vi "Cycle.vi"() -> ()   [LabVIEW 2011]
doc: "This example is a template that gives the structure of a single-loop PID controller. This VI uses the PID Filter VI to reduce measurement noise. This VI also uses the PID Autotuning VI to tune the controller based on the closed-loop response. This VI also uses the Timed Loop to ensure deterministic execution.\n\nReplace the Dummy Input and Dummy Output VIs with code that communicates with a real-time target."
uses:
  <vilib>/Platform/TimedLoop/XDataNode/timing_clust.ctl
  <vilib>/Platform/TimedLoop/XDataNode/nitl_modes.ctl
  <vilib>/Platform/TimedLoop/XDataNode/wakeup.ctl
  <vilib>/DAQmx/write.llb/DAQmx Write (Digital 1D Bool NChan 1Samp 1Line).vi
  <vilib>/DAQmx/write.llb/DAQmx Write (Counter Frequency 1Chan 1Samp).vi
  <vilib>/DAQmx/create/channels.llb/DAQmx Create Channel (CO-Pulse Generation-Frequency).vi
  <vilib>/DAQmx/configure/timing.llb/DAQmx Timing (Implicit).vi
  <vilib>/DAQmx/miscellaneous.llb/DAQmx Fill In Error Info.vi
  <vilib>/Platform/TimedLoop/XDataNode/XDataNode.xnode
  <vilib>/Platform/TimedLoop/XDataNode/XDNodeRunTimeDep.lvlib
panel:
  in  "duty cycle":dbl=0.8 format="%_6g"
  in  "Period":i64=1000
  in  "Switch":bool
  in  "stop 2":bool
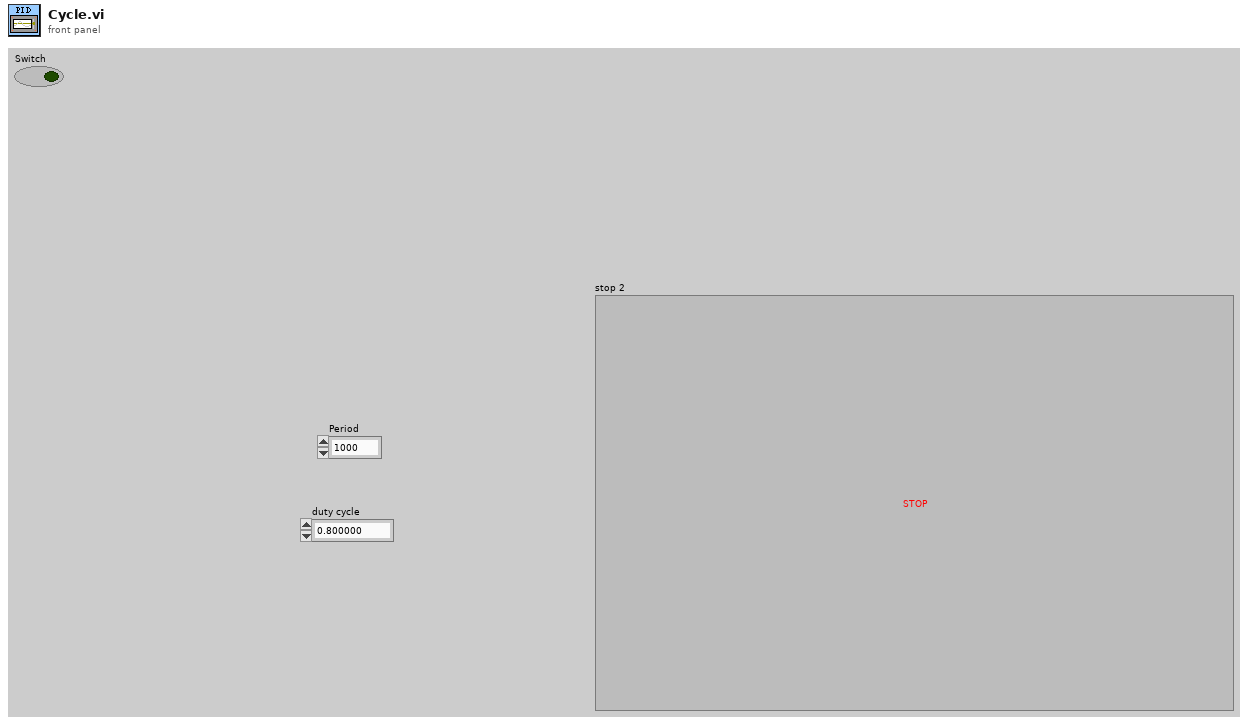
[diagram p1: front panel]
types:
  T1 = typedef "XDNodeRunTimeDep.lvlib/timing_clust.ctl" = cluster{"Expected End [f-1]":u64, "Actual End [f-1]":u64, "Finished Late? [f-1]":bool, "Expected End [i-1]":u64, "Actual End [i-1]":u64, "Finished Late? [i-1]":bool, "Expected Start [i]":u64, "Actual Start [i]":u64, "Expected Start [f]":u64, "Actual Start [f]":u64, "Source Name":string, "Structure Name":string, "Period":i64, "Deadline":i64, "Offset":i64, "Start":i64, "Priority":i32, "Timeout":i32, "Mode":T2, "Wakeup Reason":T3, "Error":errorcluster, "Source Type":string, "Secondary Source Type":string, "Global End Time":u64, "Global Start Time":u64, "Frame Duration":u64, "Iteration Duration":u64, "Assigned CPU":i32, "I/O Scan Engine Mode":u32}
  T2 = typedef "XDNodeRunTimeDep.lvlib/nitl_modes.ctl" = enum32{"No Change", "Process missed periods, maintain original phase", "Discard missed periods, maintain original phase", "Process missed periods, ignore original phase", "Discard missed periods, ignore original phase"}
  T3 = typedef "XDNodeRunTimeDep.lvlib/wakeup.ctl" = enum32{"Normal", "Aborted", "Asynchronous wakeup", "Timing source error", "Timed loop error", "Timeout"}
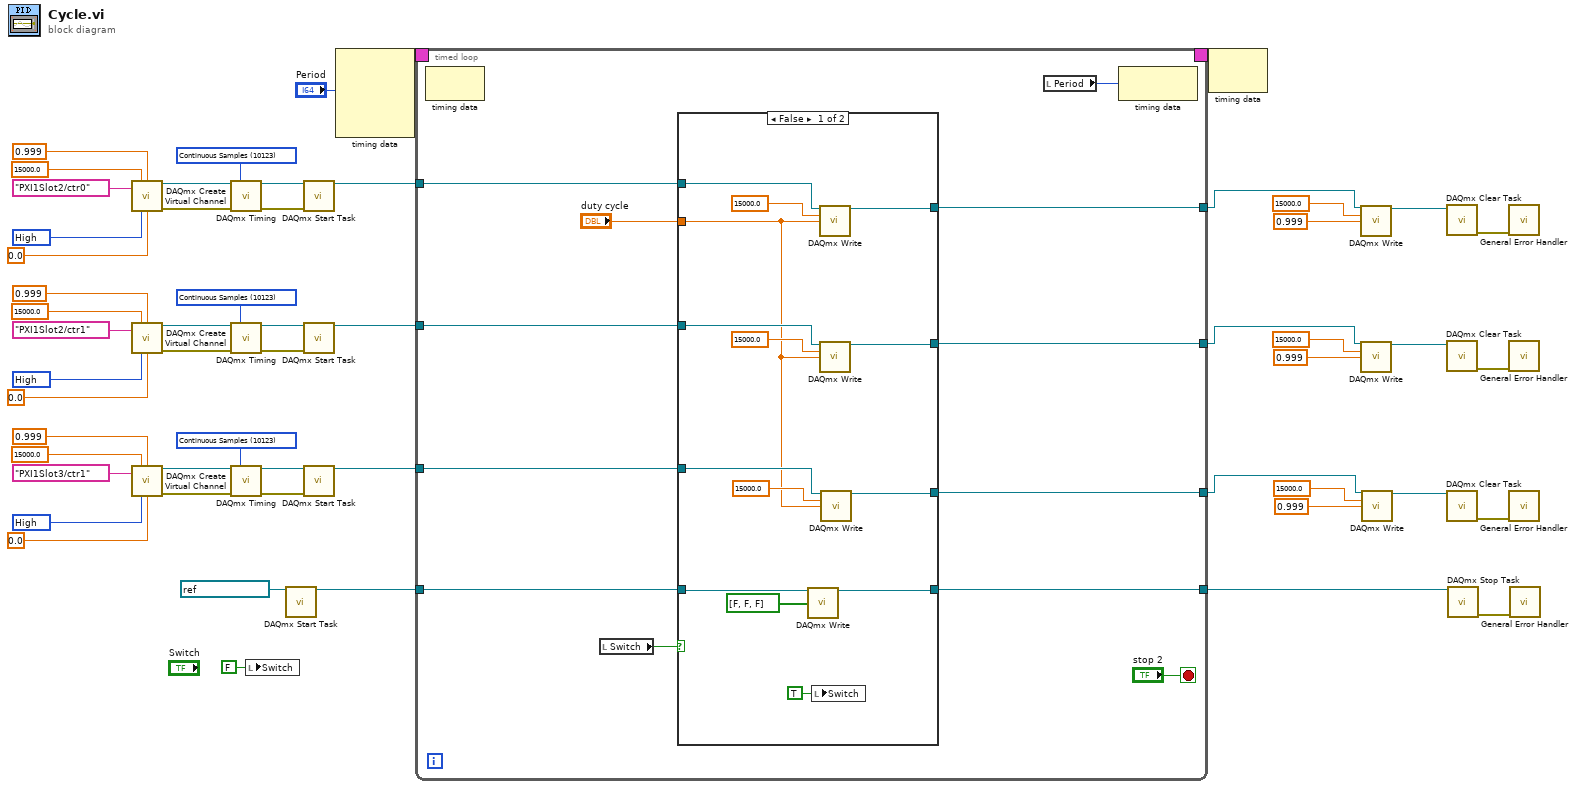
[diagram p0: block diagram]
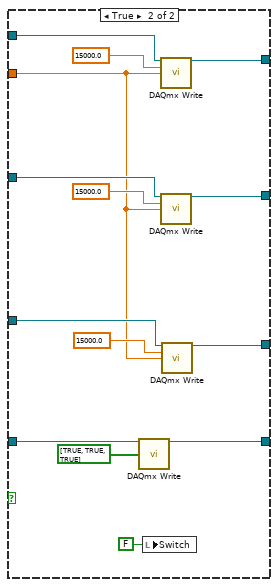
[diagram p2: hidden frame]
diagram:
  w48 = 10192 items=["High"=10192, "Low"=10214] ("idle state")
  w54 = 10123 items=["Finite Samples"=10178, "Continuous Samples"=10123] ("sample mode")
  w41 = 10192 items=["High"=10192, "Low"=10214] ("idle state")
  w35 = 10123 items=["Finite Samples"=10178, "Continuous Samples"=10123] ("sample mode")
  w28 = 10192 items=["High"=10192, "Low"=10214] ("idle state")
  w34 = 10123 items=["Finite Samples"=10178, "Continuous Samples"=10123] ("sample mode")
  n1 = call-poly <vilib>:"DAQmx Create Virtual Channel.vi"("frequency"=15000.0 ("duty cycle"), "duty cycle"=0.999, "counter"=tag "PXI1Slot2/ctr0", "idle state"=w28, "initial delay"=0.0) -> ("task out"=w31:refnum<k21>, "error out"=w30:errorcluster)  [unwired: 9 in]
  n2 = call-poly <vilib>:"DAQmx Create Virtual Channel.vi"("frequency"=15000.0 ("duty cycle"), "duty cycle"=0.999, "counter"=tag "PXI1Slot2/ctr1", "idle state"=w41, "initial delay"=0.0) -> ("task out"=w38:refnum<k21>, "error out"=w39:errorcluster)  [unwired: 9 in]
  n3 = call-poly <vilib>:"DAQmx Create Virtual Channel.vi"("frequency"=15000.0 ("duty cycle"), "duty cycle"=0.999, "counter"=tag "PXI1Slot3/ctr1", "idle state"=w48, "initial delay"=0.0) -> ("task out"=w51:refnum<k21>, "error out"=w50:errorcluster)  [unwired: 9 in]
  n4 = call-poly <vilib>:"DAQmx Timing.vi"("task/channels in"=w31, "sample mode"=w34, "error in"=w30) -> ("task out"=w33:refnum<k21>, "error out"=w32:errorcluster)  [unwired: 11 in]
  n5 = call-poly <vilib>:"DAQmx Timing.vi"("task/channels in"=w38, "sample mode"=w35, "error in"=w39) -> ("task out"=w36:refnum<k21>, "error out"=w37:errorcluster)  [unwired: 11 in]
  n6 = call-poly <vilib>:"DAQmx Timing.vi"("task/channels in"=w51, "sample mode"=w54, "error in"=w50) -> ("task out"=w53:refnum<k21>, "error out"=w52:errorcluster)  [unwired: 11 in]
  n7 = local write "Switch"(FALSE ("Switch")) -> ()
  n8 = call <vilib>:"DAQmx Start Task.vi"("task/channels in"=refnum<k21> "MotorDirABC") -> ("task out"=w16:refnum<k21>)  [unwired: 13 in, 1 out]
  n9 = call <vilib>:"DAQmx Start Task.vi"("task/channels in"=w33, "error in"=w32) -> ("task out"=w21:refnum<k21>)  [unwired: 12 in, 1 out]
  n10 = call <vilib>:"DAQmx Start Task.vi"("task/channels in"=w36, "error in"=w37) -> ("task out"=w20:refnum<k21>)  [unwired: 12 in, 1 out]
  n11 = call <vilib>:"DAQmx Start Task.vi"("task/channels in"=w53, "error in"=w52) -> ("task out"=w19:refnum<k21>)  [unwired: 12 in, 1 out]
  n12 = node-c288("Period") -> (w56:T1)  [unwired: 3 in]
  n13 = timed-loop {
    timing: w56 -> [_]
    timing-out: [_] -> w55
    tunnel: w21 -> [w68]
    tunnel: w20 -> [w67]
    tunnel: w19 -> [w66]
    tunnel: [w64] -> w5
    tunnel: [w63] -> w6
    tunnel: [w62] -> w7
    tunnel: w16 -> [w61]
    tunnel: [w60] -> w15
    stop <- "stop 2" stop-if-true
    n14 = node-c288() -> ()  [unwired: 1 in, 1 out]
    n15 = local read "Switch"() -> (w59:bool)
    n16 = case shown="False" w59 {
      tunnel: w68 -> [w70 w89]
      tunnel: w67 -> [w75 w87]
      tunnel: w66 -> [w73 w85]
      tunnel: [w69 w88] -> w64
      tunnel: [w74 w86] -> w63
      tunnel: [w72 w84] -> w62
      tunnel: w61 -> [w79 w96]
      tunnel: [w80 w95] -> w60
      tunnel: "duty cycle" -> [w71 w83]
      frame False {
        n17 = call-poly <vilib>:"DAQmx Write.vi"("task/channels in"=w79, "data"=bool[] [FALSE, FALSE, FALSE]) -> ("task out"=w80:refnum<k21>)  [unwired: 11 in, 2 out]
        n18 = local write "Switch"(TRUE ("Switch")) -> ()
        n19 = call-poly <vilib>:"DAQmx Write.vi"("task/channels in"=w70, "frequency"=15000.0, "duty cycle"=w71) -> ("task out"=w69:refnum<k21>)  [unwired: 10 in, 2 out]
        n20 = call-poly <vilib>:"DAQmx Write.vi"("task/channels in"=w75, "frequency"=15000.0, "duty cycle"=w71) -> ("task out"=w74:refnum<k21>)  [unwired: 10 in, 2 out]
        n21 = call-poly <vilib>:"DAQmx Write.vi"("task/channels in"=w73, "frequency"=15000.0, "duty cycle"=w71) -> ("task out"=w72:refnum<k21>)  [unwired: 10 in, 2 out]
      }
      frame True {
        n22 = call-poly <vilib>:"DAQmx Write.vi"("task/channels in"=w96, "data"=bool[] [TRUE, TRUE, TRUE]) -> ("task out"=w95:refnum<k21>)  [unwired: 11 in, 2 out]
        n23 = local write "Switch"(FALSE ("Switch")) -> ()
        n24 = call-poly <vilib>:"DAQmx Write.vi"("task/channels in"=w89, "frequency"=15000.0, "duty cycle"=w83) -> ("task out"=w88:refnum<k21>)  [unwired: 10 in, 2 out]
        n25 = call-poly <vilib>:"DAQmx Write.vi"("task/channels in"=w87, "frequency"=15000.0, "duty cycle"=w83) -> ("task out"=w86:refnum<k21>)  [unwired: 10 in, 2 out]
        n26 = call-poly <vilib>:"DAQmx Write.vi"("task/channels in"=w85, "frequency"=15000.0, "duty cycle"=w83) -> ("task out"=w84:refnum<k21>)  [unwired: 10 in, 2 out]
      }
    }
    n27 = local read "Period"() -> (w58:i64)
    n28 = node-c288(w58) -> ()  [unwired: 1 out]
  }
  n29 = node-c288(w55) -> ()  [unwired: 1 out]
  n30 = call-poly <vilib>:"DAQmx Write.vi"("task/channels in"=w5, "frequency"=15000.0, "duty cycle"=0.999) -> ("task out"=w4:refnum<k21>)  [unwired: 10 in, 2 out]
  n31 = call-poly <vilib>:"DAQmx Write.vi"("task/channels in"=w6, "frequency"=15000.0, "duty cycle"=0.999) -> ("task out"=w3:refnum<k21>)  [unwired: 10 in, 2 out]
  n32 = call-poly <vilib>:"DAQmx Write.vi"("task/channels in"=w7, "frequency"=15000.0, "duty cycle"=0.999) -> ("task out"=w2:refnum<k21>)  [unwired: 10 in, 2 out]
  n33 = call <vilib>:"DAQmx Clear Task.vi"("task in"=w4) -> ("error out"=w22:errorcluster)  [unwired: 14 in]
  n34 = call <vilib>:"DAQmx Clear Task.vi"("task in"=w3) -> ("error out"=w23:errorcluster)  [unwired: 14 in]
  n35 = call <vilib>:"DAQmx Clear Task.vi"("task in"=w2) -> ("error out"=w24:errorcluster)  [unwired: 14 in]
  n36 = call <vilib>:"DAQmx Stop Task.vi"("task/channels in"=w15) -> ("error out"=w17:errorcluster)  [unwired: 13 in, 1 out]
  n37 = call <vilib>:"General Error Handler.vi"("error in (no error)"=w22) -> ()  [unwired: 10 in, 5 out]
  n38 = call <vilib>:"General Error Handler.vi"("error in (no error)"=w23) -> ()  [unwired: 10 in, 5 out]
  n39 = call <vilib>:"General Error Handler.vi"("error in (no error)"=w24) -> ()  [unwired: 10 in, 5 out]
  n40 = call <vilib>:"General Error Handler.vi"("error in (no error)"=w17) -> ()  [unwired: 10 in, 5 out]
